vi "Test Status.vi"(0 "LinV2 läuft":bool, 5 "HovaCAL Interference läuft":bool, 7 "Interference 366 läuft":bool, 9 "Interference 375 läuft":bool, 11 "error in (no error)":errorcluster caption="Fehler (Eingang, kein Fehler)", 13 "Aktion":T2) -> (4 "String":string, 8 "Aktive Tests":T1, 10 "Tests sperren":bool, 15 "error out":errorcluster caption="Fehler (Ausgang)")   [LabVIEW 2020, in "EPA 1065.lvlib"]
uses:
  EPA 1065.lvlib
  Aktion Test Status.ctl
  Aktive Tests Cluster.ctl
  Sprachverwaltung/FGV Aktion Tabelle zerlegen.ctl
  T90 1065-308/Aktion FGV T90.ctl
  Dichtheitstest 1065-345/Aktion Leak Daten.ctl
  Sprachverwaltung/Sprachverwaltung.lvlib
  ANR Test 1065-305/ARN Test 1065-305.lvlib
  T90 1065-308/T90 Test 1065-308.lvlib
  Dichtheitstest 1065-345/Dichtheitstest 1065-345.lvlib
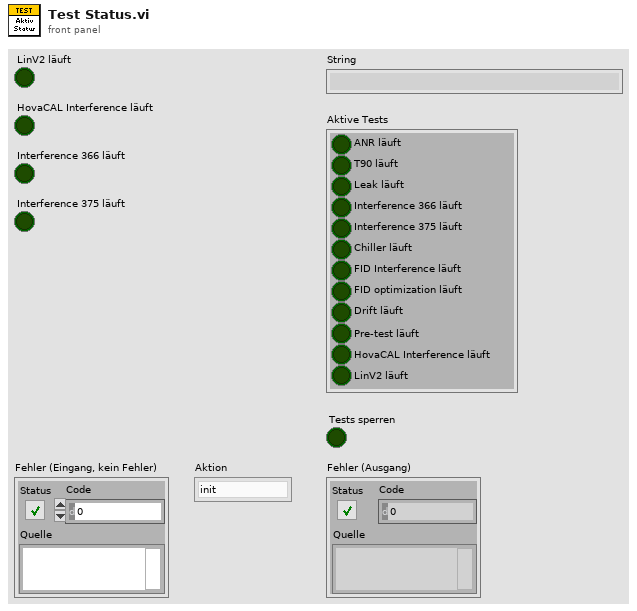
[diagram p1: front panel]
types:
  T1 = typedef "EPA 1065.lvlib/Aktive Tests Cluster.ctl" = cluster{"ANR läuft":bool, "T90 läuft":bool, "Leak läuft":bool, "Interference 366 läuft":bool, "Interference 375 läuft":bool, "Chiller läuft":bool, "FID Interference läuft":bool, "FID optimization läuft":bool, "Drift läuft":bool, "Pre-test läuft":bool, "HovaCAL Interference läuft":bool, "LinV2 läuft":bool}
  T2 = typedef "EPA 1065.lvlib/Aktion Test Status.ctl" = enum16{"init", "lesen", "prüfen", "Interference 366", "Interference 375", "Chiller läuft", "Drift läuft", "Pre Test läuft", "FID Optimization läuft", "FID Interference läuft", "HovaCAL Interference", "LinV2"}
  T3 = typedef "Sprachverwaltung.lvlib/FGV Aktion Tabelle zerlegen.ctl" = enum16{"laden", "vereinzeln", "speichern"}
  T4 = typedef "EPA 1065.lvlib/Dichtheitstest 1065-345.lvlib/Aktion Leak Daten.ctl" = enum16{"lesen", "laden", "speichern", "Volumen", "berechnen", "Leak check aktiv", "Leak Zustand", "Pfad", "Pfad speichern"}
  T5 = typedef "EPA 1065.lvlib/T90 Test 1065-308.lvlib/Aktion FGV T90.ctl" = enum16{"lesen", "Konfig Daten", "speichern", "laden", "T90 aktiv", "T90 inaktiv", "Ext. Ventil aktivieren", "Ext. Ventil deaktivieren", "N2 spülen aktiv", "N2 spülen inaktiv", "Ergebnis Textfile"}
  T6 = enum16{"init", "lesen", "ARN Test aktiv", "ARN Test inaktiv"}
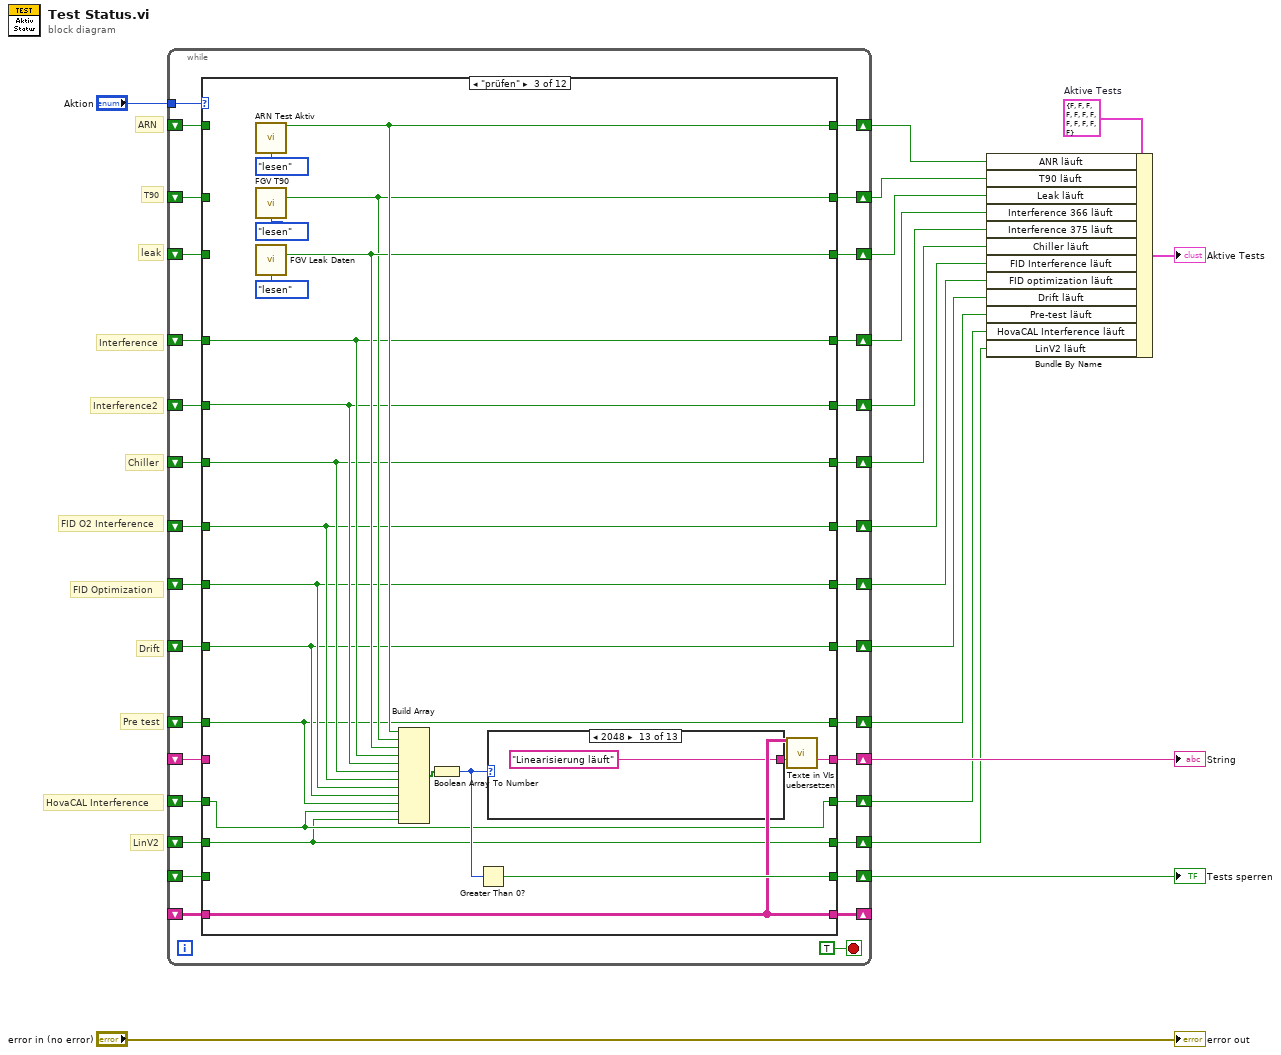
[diagram p0: block diagram]
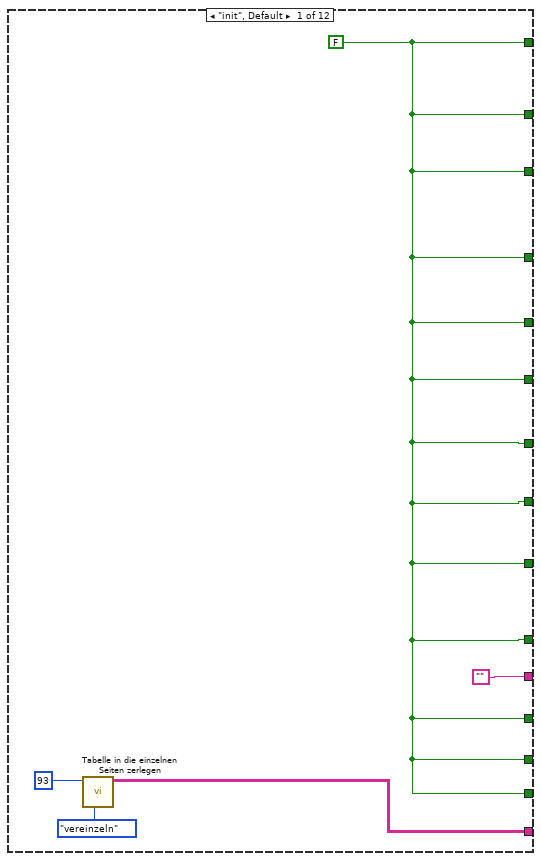
[diagram p2: hidden frame]
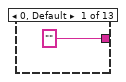
[diagram p4: hidden frame]
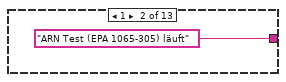
[diagram p5: hidden frame]
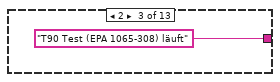
[diagram p6: hidden frame]
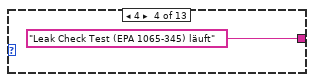
[diagram p7: hidden frame]
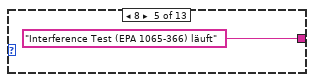
[diagram p8: hidden frame]
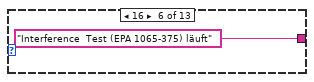
[diagram p9: hidden frame]
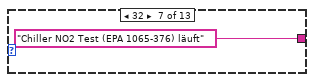
[diagram p10: hidden frame]
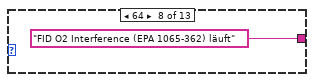
[diagram p11: hidden frame]
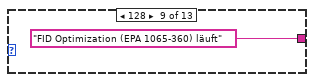
[diagram p12: hidden frame]
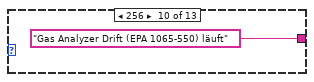
[diagram p13: hidden frame]
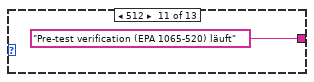
[diagram p14: hidden frame]
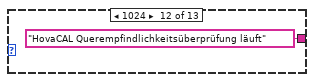
[diagram p15: hidden frame]
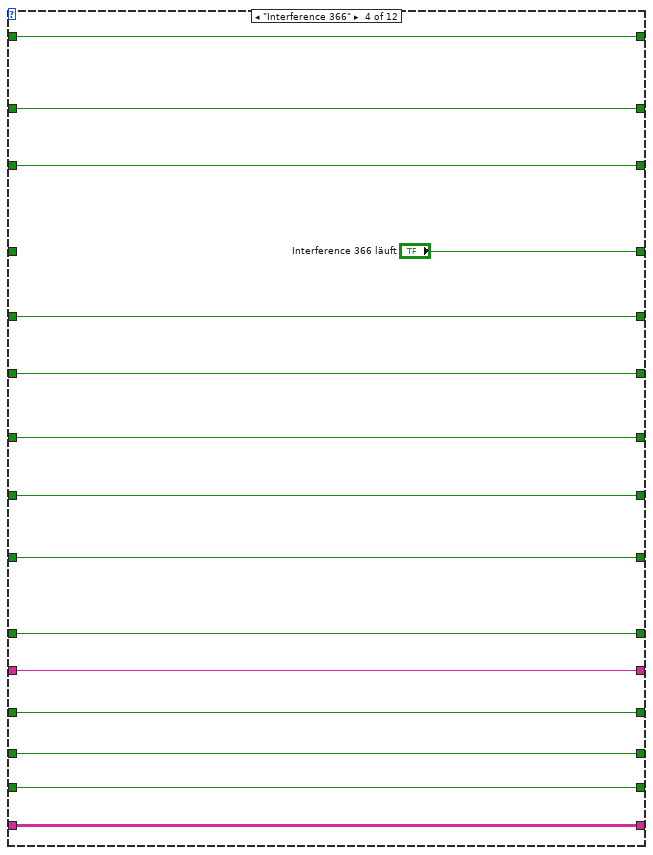
[diagram p16: hidden frame]
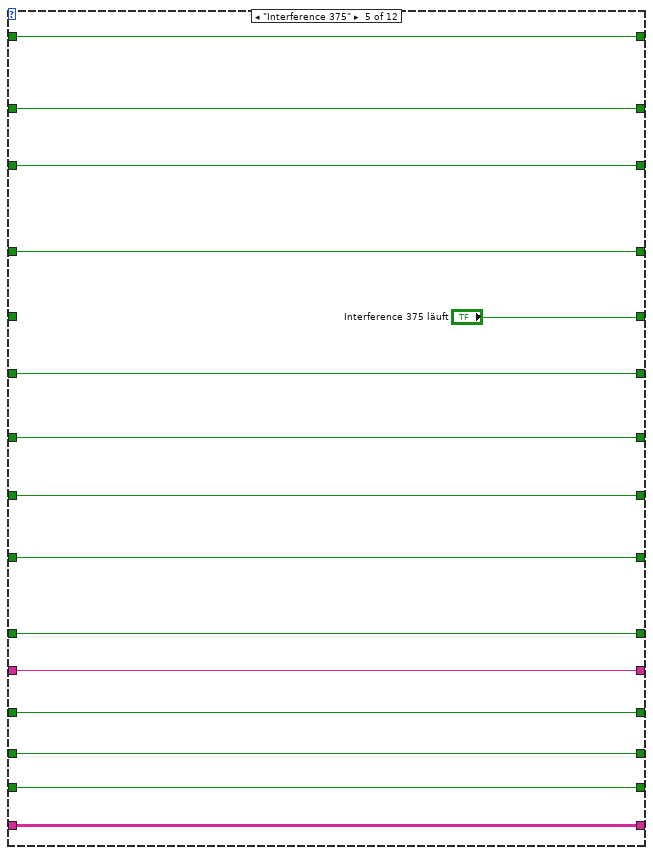
[diagram p17: hidden frame]
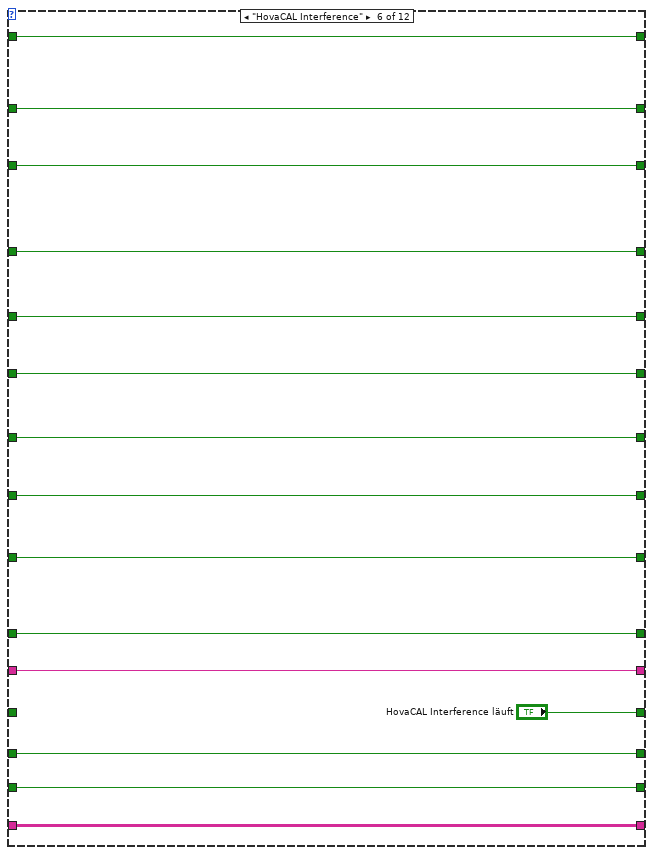
[diagram p18: hidden frame]
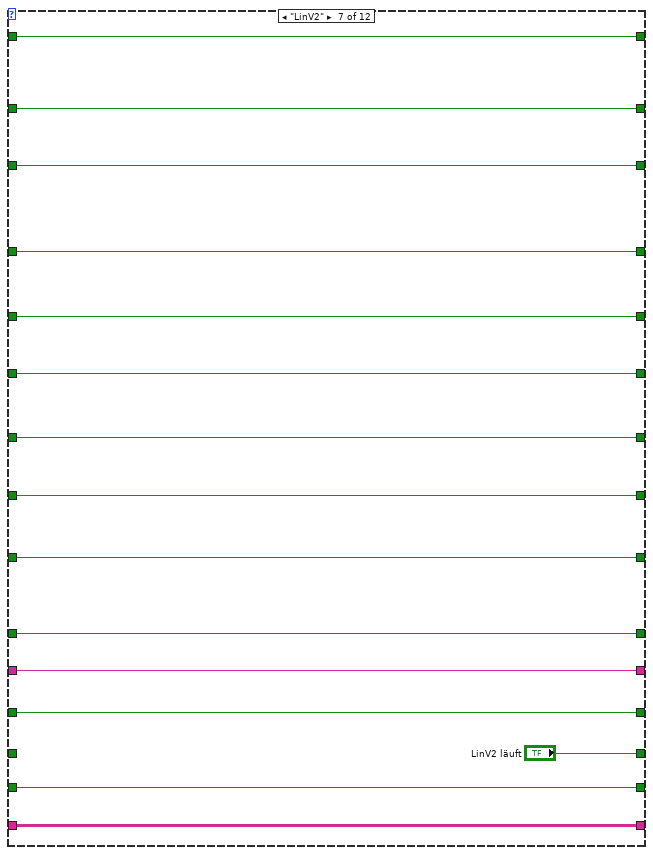
[diagram p19: hidden frame]
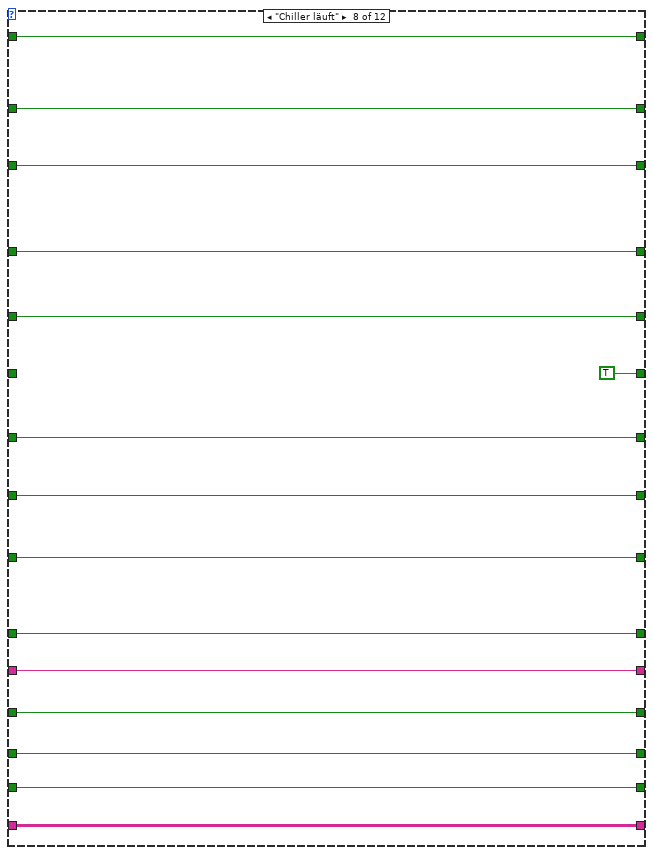
[diagram p20: hidden frame]
diagram:
  w15 = T1 {"ANR läuft"=FALSE, "T90 läuft"=FALSE, "Leak läuft"=FALSE, "Interference 366 läuft"=FALSE, "Interference 375 läuft"=FALSE, "Chiller läuft"=FALSE, "FID Interference läuft"=FALSE, "FID optimization läuft"=FALSE, "Drift läuft"=FALSE, "Pre-test läuft"=FALSE, "HovaCAL Interference läuft"=FALSE, "LinV2 läuft"=FALSE}  # Aktive Tests
  # "LinV2"
  # "HovaCAL Interference"
  # "Pre test"
  # "Drift"
  # "FID Optimization"
  # "FID O2 Interference"
  # "Chiller"
  # "Interference2"
  # "Interference"
  # "leak"
  # "T90"
  # "ARN"
  n1 = while {
    tunnel: "Aktion" -> [w49]
    shift-right: [w48] -> w14
    shift-left: _ -> [w47]
    shift-right: [w46] -> w13
    shift-left: _ -> [w45]
    shift-right: [w44] -> w12
    shift-left: _ -> [w43]
    shift-right: [w41] -> w11
    shift-left: _ -> [w40]
    shift-right: [w39] -> w10
    shift-left: _ -> [w38]
    shift-right: [w36] -> _
    shift-left: _ -> [w35]
    shift-right: [w37] -> w16
    shift-left: _ -> [w34]
    shift-right: [w42] -> w17
    shift-left: _ -> [w33]
    shift-right: [w32] -> w8
    shift-left: _ -> [w31]
    shift-right: [w29] -> w7
    shift-left: _ -> [w30]
    shift-right: [w28] -> w6
    shift-left: _ -> [w27]
    shift-right: [w25] -> w5
    shift-left: _ -> [w26]
    shift-right: [w24] -> w4
    shift-left: _ -> [w23]
    shift-right: [w22] -> w3
    shift-left: _ -> [w21]
    shift-right: [w20] -> w1
    shift-left: _ -> [w19]
    stop <- TRUE stop-if-true
    n2 = case shown="\"prüfen\"" w49 {
      tunnel: [w51 w68 w82 w112 w127 w143 w158 w179 w194 w209 w224 w239] -> w48
      tunnel: w47 -> [_ w68 _ w112 w127 w143 w158 w179 w194 w209 w224 w239]
      tunnel: [w51 w67 w80 w113 w128 w144 w159 w178 w193 w208 w223 w238] -> w46
      tunnel: w45 -> [_ w67 _ w113 w128 w144 w159 w178 w193 w208 w223 w238]
      tunnel: [w51 w66 w81 w114 w129 w145 w160 w177 w192 w207 w222 w237] -> w44
      tunnel: w43 -> [_ w66 _ w114 w129 w145 w160 w177 w192 w207 w222 w237]
      tunnel: ["" w63 w87 w115 w130 w146 w161 w176 w191 w206 w221 w236] -> w42
      tunnel: [w51 w65 w79 "Interference 366 läuft" w132 w147 w162 w175 w190 w205 w220 w235] -> w41
      tunnel: w40 -> [_ w65 w79 _ w132 w147 w162 w175 w190 w205 w220 w235]
      tunnel: [w51 w64 w78 w116 "Interference 375 läuft" w137 w152 w174 w189 w204 w219 w234] -> w39
      tunnel: w38 -> [_ w64 w78 w116 _ w137 w152 w174 w189 w204 w219 w234]
      tunnel: [w51 w69 w89 w119 w134 w149 w164 w173 w188 w203 w218 w233] -> w37
      tunnel: [w53 w70 w86 w118 w133 w148 w163 w172 w187 w202 w217 w232] -> w36
      tunnel: w35 -> [_ w70 w86 w118 w133 w148 w163 w172 w187 w202 w217 w232]
      tunnel: w34 -> [_ w69 _ w119 w134 w149 w164 w173 w188 w203 w218 w233]
      tunnel: w33 -> [_ w63 _ w115 w130 w146 w161 w176 w191 w206 w221 w236]
      tunnel: [w51 w62 w77 w111 w126 w142 w157 TRUE w186 w201 w216 w231] -> w32
      tunnel: w31 -> [_ w62 w77 w111 w126 w142 w157 _ w186 w201 w216 w231]
      tunnel: [w51 w61 w76 w110 w125 w141 w156 w171 w185 w200 w215 TRUE] -> w29
      tunnel: w30 -> [_ w61 w76 w110 w125 w141 w156 w171 w185 w200 w215 _]
      tunnel: [w51 w60 w75 w109 w124 w140 w155 w170 w184 w199 TRUE w230] -> w28
      tunnel: w27 -> [_ w60 w75 w109 w124 w140 w155 w170 w184 w199 _ w230]
      tunnel: [w51 w59 w74 w108 w123 w139 w154 w169 TRUE w198 w214 w229] -> w25
      tunnel: w26 -> [_ w59 w74 w108 w123 w139 w154 w169 _ w198 w214 w229]
      tunnel: [w51 w58 w73 w107 w122 w138 w153 w168 w183 TRUE w213 w228] -> w24
      tunnel: w23 -> [_ w58 w73 w107 w122 w138 w153 w168 w183 _ w213 w228]
      tunnel: [w51 w57 w72 w106 w121 "HovaCAL Interference läuft" w151 w166 w181 w196 w211 w226] -> w22
      tunnel: w21 -> [_ w57 w72 w106 w121 _ w151 w166 w181 w196 w211 w226]
      tunnel: [w51 w56 w71 w105 w120 w135 "LinV2 läuft" w165 w180 w195 w210 w225] -> w20
      tunnel: w19 -> [_ w56 w71 w105 w120 w135 _ w165 w180 w195 w210 w225]
      frame "init", Default {
        w51 = FALSE
        n3 = call "Tabelle in die einzelnen Seiten zerlegen.vi"("Aktion"=FGV_Aktion_Tabelle_zerlegen."vereinzeln", "Index (Seite)"=93) -> ("Sprachliste"=w53:string[][])  [unwired: 7 in, 2 out]
      }
      frame "lesen" {
      }
      frame "prüfen" {
        n4 = call "ARN Test Aktiv.vi"("Aktion"=T6."lesen") -> ("ARN Test Aktiv"=w82:bool)  [unwired: 13 in, 1 out]
        n5 = call "FGV T90.vi"("Aktion"=Aktion_FGV_T90."lesen") -> ("T90 Aktiv"=w80:bool)  [unwired: 9 in, 5 out]
        n6 = call "FGV Leak Daten.vi"("Aktion"=Aktion_Leak_Daten."lesen") -> ("Dichtheitstest aktiv"=w81:bool)  [unwired: 10 in, 4 out]
        n7 = Build Array(w82, w80, w81, w79, w78, w77, w76, w75, w74, w73, w72, w71) -> (w91:bool[])
        n8 = Boolean Array To Number(Boolean array=w91) -> (number=w90:u32)
        n9 = Greater Than 0?(x=w90) -> (x > 0?=w89:bool)
        n10 = case shown="2048" w90 {
          tunnel: ["" "ARN Test (EPA 1065-305) läuft" "T90 Test (EPA 1065-308) läuft" "Leak Check Test (EPA 1065-345) läuft" "Interference Test (EPA 1065-366) läuft" "Interference  Test (EPA 1065-375) läuft" "Chiller NO2 Test (EPA 1065-376) läuft" "FID O2 Interference (EPA 1065-362) läuft" "FID Optimization (EPA 1065-360) läuft" "Gas Analyzer Drift (EPA 1065-550) läuft" "Pre-test verification (EPA 1065-520) läuft" "HovaCAL Querempfindlichkeitsüberprüfung läuft" "Linearisierung läuft"] -> w88
          frame 0, Default {
          }
          frame 1 {
          }
          frame 2 {
          }
          frame 4 {
          }
          frame 8 {
          }
          frame 16 {
          }
          frame 32 {
          }
          frame 64 {
          }
          frame 128 {
          }
          frame 256 {
          }
          frame 512 {
          }
          frame 1024 {
          }
          frame 2048 {
          }
        }
        n11 = call "Texte in VIs uebersetzen.vi"("Sprachliste"=w86, "String zum Übersetzen"=w88) -> ("String zum Übersetzen"=w87:string)  [unwired: 9 in, 4 out]
      }
      frame "Interference 366" {
      }
      frame "Interference 375" {
      }
      frame "HovaCAL Interference" {
      }
      frame "LinV2" {
      }
      frame "Chiller läuft" {
      }
      frame "Drift läuft" {
      }
      frame "Pre Test läuft" {
      }
      frame "FID Optimization läuft" {
      }
      frame "FID Interference läuft" {
      }
    }
  }
  "String" <- w17
  "Tests sperren" <- w16
  n12 = Bundle By Name(cluster=w15, "ANR läuft"=w14, "T90 läuft"=w13, "Leak läuft"=w12, "Interference 366 läuft"=w11, "Interference 375 läuft"=w10, "Chiller läuft"=w8, "FID Interference läuft"=w7, "FID optimization läuft"=w6, "Drift läuft"=w5, "Pre-test läuft"=w4, "HovaCAL Interference läuft"=w3, "LinV2 läuft"=w1) -> (→"Aktive Tests":T1)
  "error out" <- "error in (no error)"
